vi "DropDetection ver 4.vi"(8 "error in":errorcluster, 11 "Path":path) -> (0 "error out":errorcluster, 1 "Image Out":T1(plugin-control), 2 "Particle Measurements (Pixels)":dbl[][](array[numeric]) format="%.2f", 3 "Number of Particles":i32)   [LabVIEW 2013]
uses:
  <vilib>/vision/NI_Vision_Development_Module.lvlib
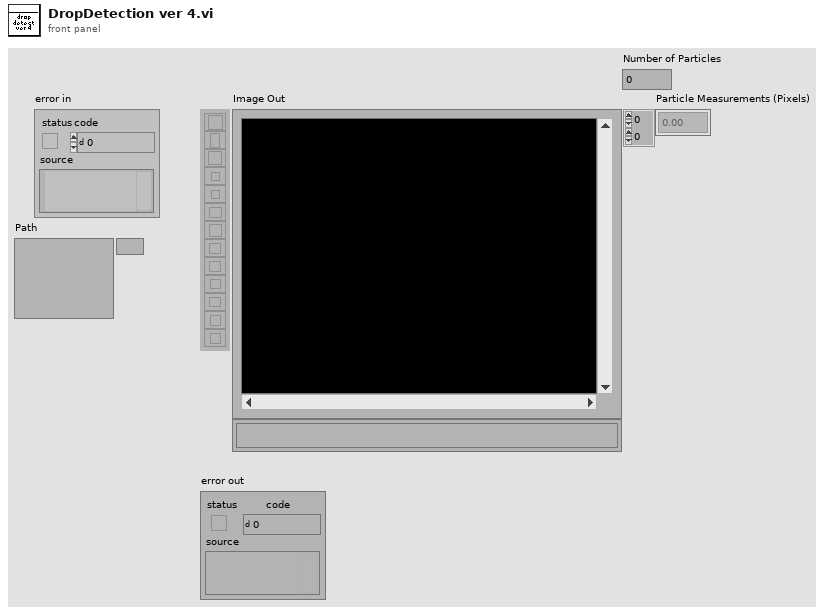
[diagram p1: front panel]
types:
  T1 = typedef "IMAQ Image.ctl" = refnum<image>
  T2 = enum32{"AutoM", "Close", "Dilate", "Erode", "Gradient", "Gradient out", "Gradient in", "Hit miss", "Open", "PClose", "POpen", "Thick", "Thin"}
  T3 = cluster{"Registration Method":u32, "Normalization Method":u32, "Edge Thickness to Ignore":i32, "Bright Threshold":sgl, "Dark Threshold":sgl, "Grayscale/ Binary?":bool}
  T4 = typedef "Image Type" = u32
  T5 = cluster{"Transformed point":cluster{"Left":sgl, "Top":sgl}, "Transformed Angle":sgl, "Numeric out":dbl}
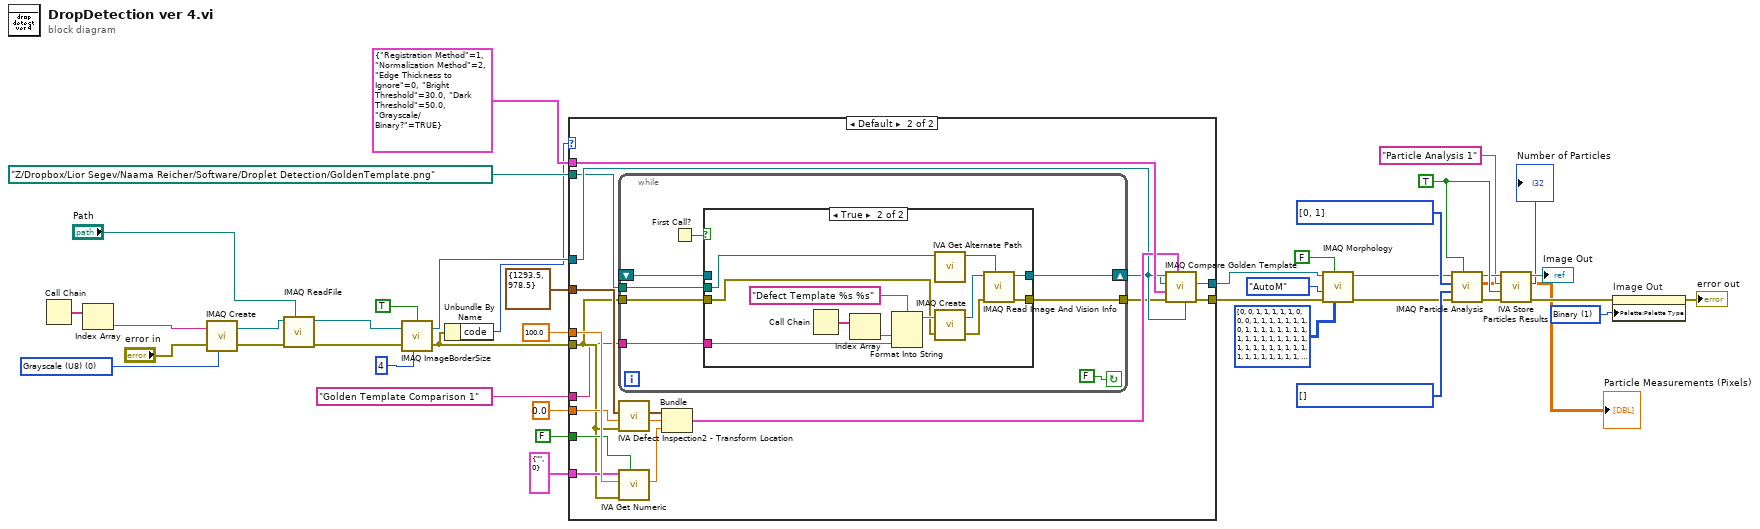
[diagram p0: block diagram]
diagram:
  w6 = u32 1 items=["Grayscale", "Binary", "Gradient", "Rainbow", "Temperature", "User Defined"] ("Palette")
  w14 = i32[] [] items=["Center of Mass X", "Center of Mass Y", "First Pixel X", "First Pixel Y", "Bounding Rect Left", "Bounding Rect Top", "Bounding Rect Right", "Bounding Rect Bottom", "Max Feret Diameter Start X", "Max Feret Diameter Start Y", "Max Feret Diameter End X", "Max Feret Diameter End Y", "Max Horiz. Segment Length Left", "Max Horiz. Segment Length Right", "Max Horiz. Segment Length Row", "-", "Bounding Rect Width", "Bounding Rect Height", "Bounding Rect Diagonal", "Perimeter", "Convex Hull Perimeter", "Holes' Perimeter", "Max Feret Diameter", "Equivalent Ellipse Major Axis", "Equivalent Ellipse Minor Axis", "Equivalent Ellipse Minor Axis (Feret)", "Equivalent Rect Long Side", "Equivalent Rect Short Side", "Equivalent Rect Diagonal", "Equivalent Rect Short Side (Feret)", "Average Horiz. Segment Length", "Average Vert. Segment Length", "Hydraulic Radius", "Waddel Disk Diameter", "-", "Area", "Holes' Area", "Particle & Holes' Area", "Convex Hull Area", "Image Area", "-", "Number of Holes", "Number of Horiz. Segments", "Number of Vert. Segments", "-", "Orientation", "Max Feret Diameter Orientation", "-", "% Area/Image Area", "% Area/(Particle & Holes' Area)", "Ratio of Equivalent Ellipse Axes", "Ratio of Equivalent Rect Sides", "-", "Elongation Factor", "Compactness Factor", "Heywood Circularity Factor", "Type Factor", "-", "Sum X", "Sum Y", "Sum XX", "Sum XY", "Sum YY", "Sum XXX", "Sum XXY", "Sum XYY", "Sum YYY", "-", "Moment of Inertia XX", "Moment of Inertia XY", "Moment of Inertia YY", "Moment of Inertia XXX", "Moment of Inertia XXY", "Moment of Inertia XYY", "Moment of Inertia YYY", "Norm. Moment of Inertia XX", "Norm. Moment of Inertia XY", "Norm. Moment of Inertia YY", "Norm. Moment of Inertia XXX", "Norm. Moment of Inertia XXY", "Norm. Moment of Inertia XYY", "Norm. Moment of Inertia YYY", "Hu Moment 1", "Hu Moment 2", "Hu Moment 3", "Hu Moment 4", "Hu Moment 5", "Hu Moment 6", "Hu Moment 7"] ("Real-World Measurements")
  w15 = i32[] [0, 1] items=["Center of Mass X", "Center of Mass Y", "First Pixel X", "First Pixel Y", "Bounding Rect Left", "Bounding Rect Top", "Bounding Rect Right", "Bounding Rect Bottom", "Max Feret Diameter Start X", "Max Feret Diameter Start Y", "Max Feret Diameter End X", "Max Feret Diameter End Y", "Max Horiz. Segment Length Left", "Max Horiz. Segment Length Right", "Max Horiz. Segment Length Row", "-", "Bounding Rect Width", "Bounding Rect Height", "Bounding Rect Diagonal", "Perimeter", "Convex Hull Perimeter", "Holes' Perimeter", "Max Feret Diameter", "Equivalent Ellipse Major Axis", "Equivalent Ellipse Minor Axis", "Equivalent Ellipse Minor Axis (Feret)", "Equivalent Rect Long Side", "Equivalent Rect Short Side", "Equivalent Rect Diagonal", "Equivalent Rect Short Side (Feret)", "Average Horiz. Segment Length", "Average Vert. Segment Length", "Hydraulic Radius", "Waddel Disk Diameter", "-", "Area", "Holes' Area", "Particle & Holes' Area", "Convex Hull Area", "Image Area", "-", "Number of Holes", "Number of Horiz. Segments", "Number of Vert. Segments", "-", "Orientation", "Max Feret Diameter Orientation", "-", "% Area/Image Area", "% Area/(Particle & Holes' Area)", "Ratio of Equivalent Ellipse Axes", "Ratio of Equivalent Rect Sides", "-", "Elongation Factor", "Compactness Factor", "Heywood Circularity Factor", "Type Factor", "-", "Sum X", "Sum Y", "Sum XX", "Sum XY", "Sum YY", "Sum XXX", "Sum XXY", "Sum XYY", "Sum YYY", "-", "Moment of Inertia XX", "Moment of Inertia XY", "Moment of Inertia YY", "Moment of Inertia XXX", "Moment of Inertia XXY", "Moment of Inertia XYY", "Moment of Inertia YYY", "Norm. Moment of Inertia XX", "Norm. Moment of Inertia XY", "Norm. Moment of Inertia YY", "Norm. Moment of Inertia XXX", "Norm. Moment of Inertia XXY", "Norm. Moment of Inertia XYY", "Norm. Moment of Inertia YYY", "Hu Moment 1", "Hu Moment 2", "Hu Moment 3", "Hu Moment 4", "Hu Moment 5", "Hu Moment 6", "Hu Moment 7"] ("Pixel Measurements")
  w11 = TRUE ("Connectivity 4/8 (8)")
  w36 = T4 0 items=["Grayscale (U8)", "Grayscale (I16)", "Grayscale (SGL)", "Complex (CSG)", "RGB (U32)", "HSL (U32)", "RGB (U64)", "Grayscale (U16)"] ("Image Type")
  n1 = Call Chain() -> (call chain=w38:string[])
  n2 = Index Array(array=w38) -> (element=w37:string)  [unwired: 1 in]
  n3 = call "IMAQ Create"("Image Name"=w37, "Image Type"=w36, "error in (no error)"="error in") -> ("New Image"=w41:T1, "error out"=w40:errorcluster)  [unwired: 1 in, 1 out]
  n4 = call "IMAQ ReadFile"("File Path"="Path", "error in (no error)"=w40, "Image"=w41) -> ("error out"=w34:errorcluster, "Image Out"=w35:T1)  [unwired: 2 in, 5 out]
  n5 = call "IMAQ ImageBorderSize"("Get/Set Status? (Set)"=TRUE, "Image"=w35, "Image border size in"=4 ("Border Size"), "error in (no error)"=w34) -> ("Image Out"=w24:T1, "error out"=w23:errorcluster)  [unwired: 1 out]
  n6 = Unbundle By Name(w23) -> ("code"=w22:i32)
  n7 = case shown="Default" w22 {
    tunnel: path "Z:/Dropbox/Lior Segev/Naama Reicher/Software/Droplet Detection/GoldenTemplate.png" ("Template File Path") -> [_ w48]
    tunnel: T3 {"Registration Method"=1, "Normalization Method"=2, "Edge Thickness to Ignore"=0, "Bright Threshold"=30.0, "Dark Threshold"=50.0, "Grayscale/ Binary?"=TRUE} ("Inspection Options") -> [_ w60]
    tunnel: [_ w44] -> w16
    tunnel: [w42 w59] -> w17
    tunnel: 100.0 ("Scale") -> [_ w58]
    tunnel: cluster{"GUID":string, "Index":i32} {"GUID"="", "Index"=0} ("Scale ID") -> [_ w57]
    tunnel: FALSE ("Scale Source") -> [_ w56]
    tunnel: cluster{"x":sgl, "y":sgl} {"x"=1293.5, "y"=978.5} ("Position") -> [_ w53]
    tunnel: sgl 0.0 ("Angle") -> [_ w52]
    tunnel: w23 -> [_ w45]
    tunnel: w24 -> [w42 w49]
    tunnel: "Golden Template Comparison 1" ("Step Name") -> [_ w43]
    frame -1074396199, -1074396198 {
      # "Discard Coordinate System Error"
    }
    frame Default {
      n8 = while {
        shift-right: [w67] -> w47
        shift-left: _ -> [w66]
        tunnel: [w64] -> w46
        tunnel: w45 -> [w63]
        tunnel: w48 -> [w62]
        tunnel: w43 -> [w61]
        stop <- FALSE continue-if-true
        n9 = First Call?() -> (First Call?: T/F=w68:bool)
        n10 = case shown="True" w68 {
          tunnel: [w70 w80] -> w67
          tunnel: w66 -> [w70 _]
          tunnel: [w69 w77] -> w64
          tunnel: w63 -> [w69 w76]
          tunnel: w62 -> [_ w73]
          tunnel: w61 -> [_ w71]
          frame False {
          }
          frame True {
            n11 = Call Chain() -> (call chain=w75:string[])
            n12 = Index Array(array=w75) -> (element=w74:string)  [unwired: 1 in]
            n13 = Format Into String(format string="Defect Template %s %s" ("Image Name"), w74, w71) -> (resulting string=w82:string)  [unwired: 2 in, 1 out]
            n14 = call <vilib>:"IVA Get Alternate Path.vi"("Path In"=w73) -> ("Path Out"=w72:path)  [unwired: 10 out]
            n15 = call "IMAQ Create"("Image Name"=w82, "error in (no error)"=w76) -> ("New Image"=w79:T1, "error out"=w78:errorcluster)  [unwired: 2 in, 1 out]
            n16 = call "IMAQ Read Image And Vision Info"("File Path"=w72, "error in (no error)"=w78, "Image"=w79) -> ("error out"=w77:errorcluster, "Image Out"=w80:T1)  [unwired: 1 in, 6 out]
          }
        }
      }
      n17 = call <vilib>:"IVA Defect Inspection2 - Transform Location.vi"("error in (no error)"=w45, "Angle"=w52, "Point"=w53) -> ("Transformed Angle"=w50:sgl, "Transformed point"=w51:cluster{"Left":sgl, "Top":sgl})  [unwired: 1 in, 6 out]
      n18 = call <vilib>:"IVA Get Numeric.vi"("Source"=w56, "error in"=w45, "Numeric in"=w58, "Result ID"=w57) -> ("Numeric out"=w55:dbl)  [unwired: 7 out]
      n19 = Bundle("Transformed point"=w51, "Transformed Angle"=w50, "Numeric out"=w55) -> (w54:T5)  [unwired: 1 out]
      n20 = call "IMAQ Compare Golden Template"("Dark Defect Image Dst"=w49, "Alignment"=w54, "error in (no error)"=w46, "Inspection Options"=w60, "Template Image"=w47, "Image"=w49) -> ("error out"=w44:errorcluster, "Dark Defect Image Dst Out"=w59:T1)  [unwired: 1 in, 3 out]
    }
  }
  n21 = call "IMAQ Morphology"("Structuring Element"=i32[][] [[0, 0, 1, 1, 1, 1, 1, 0, 0], [0, 1, 1, 1, 1, 1, 1, 1, 0], [1, 1, 1, 1, 1, 1, 1, 1, 1], [1, 1, 1, 1, 1, 1, 1, 1, 1], [1, 1, 1, 1, 1, 1, 1, 1, 1], [1, 1, 1, 1, 1, 1, 1, 1, 1], [1, 1, 1, 1, 1, 1, 1, 1, 1], [0, 1, 1, 1, 1, 1, 1, 1, 0], [0, 0, 1, 1, 1, 1, 1, 0, 0]], "Square/Hexa (Square)"=FALSE, "error in (no error)"=w16, "Operation"=T2."AutoM", "Image Src"=w17) -> ("error out"=w13:errorcluster, "Image Dst Out"=w12:T1)  [unwired: 2 in, 3 out]
  n22 = call "IMAQ Particle Analysis"("Connectivity 4/8 (8)"=w11, "error in (no error)"=w13, "Real-World Measurements"=w14, "Pixel Measurements"=w15, "Image"=w12) -> ("error out"=w8:errorcluster, "Particle Measurements (Pixels)"=→"Particle Measurements (Pixels)":dbl[][], "Image Out (duplicate)"=w10:T1)  [unwired: 4 out]
  n23 = call <vilib>:"IVA Store Particles Results.vi"("error in (no error)"=w8, "Connectivity 4/8 (8)"=w11, "Step Name"="Particle Analysis 1", "Image in"=w10) -> ("error out"=w5:errorcluster, "Number of Particles"=→"Number of Particles":i32, "Image dup"=→"Image Out":T1)  [unwired: 5 out]
  n24 = property on="Image Out" class="ImageControl"(error in=w5, "Palette:Palette Type"=w6) -> (error out=→"error out":errorcluster)  [unwired: 1 in, 1 out]
